vi "Vision1.vi"   [LabVIEW 2016]
uses:
  Campbell!!!4-12/AxonCode/Robot Global Data.vi
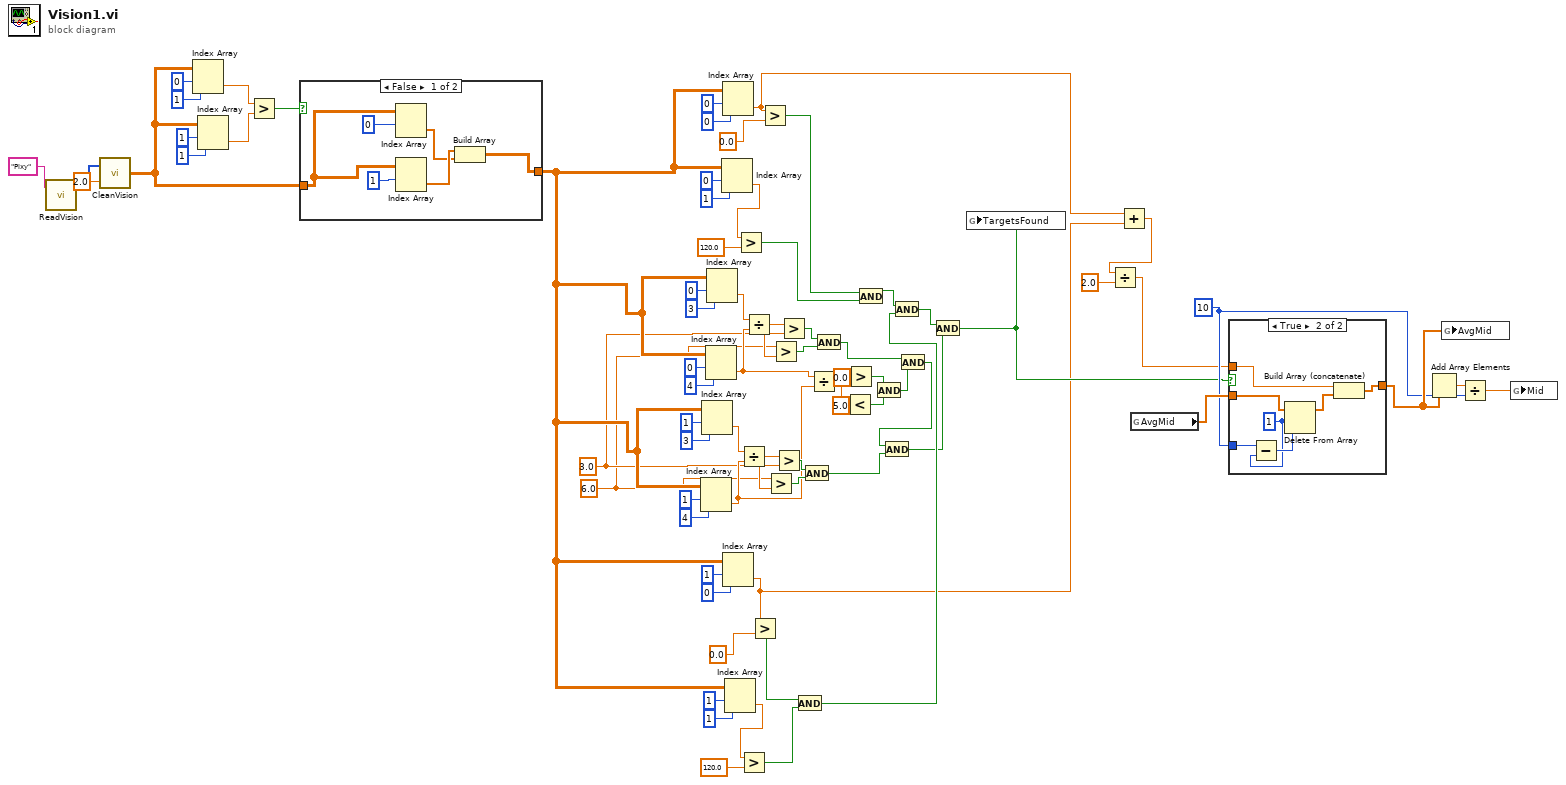
[diagram p0: block diagram]
diagram:
  w1 = 6.0 ("x")
  w2 = 3.0 ("y")
  w58 = 10
  n1 = call "ReadVision.vi"("Name"="Pixy") -> ("Target Data"=w73:u16[])  [unwired: 2 in]
  n2 = call "CleanVision.vi"("Targets"=2.0, "Input"=w73) -> ("Output"=w4:dbl[][])
  n3 = Index Array(array=w4, index (row)=0, index (col)=1 ("disabled index (col)")) -> (element=w6:dbl)
  n4 = Index Array(array=w4, index (row)=1, index (col)=1 ("disabled index (col)")) -> (element=w7:dbl)
  n5 = Greater?(x=w6, y=w7) -> (0:w5:bool)
  n6 = case shown="False" w5 {
    tunnel: w4 -> [w79 w81]
    tunnel: [w75 w81] -> w3
    frame False {
      n7 = Index Array(array=w79, index (row)=0) -> (element=w76:dbl[])  [unwired: 1 in]
      n8 = Index Array(array=w79, index (row)=1) -> (element=w77:dbl[])  [unwired: 1 in]
      n9 = Build Array(w77, w76) -> (w75:dbl[][])
    }
    frame True {
    }
  }
  n10 = Index Array(array=w3, index (row)=1, index (col)=4 ("disabled index (col)")) -> (element=w29:dbl)
  n11 = Index Array(array=w3, index (row)=1, index (col)=3 ("disabled index (col)")) -> (element=w34:dbl)
  n12 = Index Array(array=w3, index (row)=0, index (col)=4 ("disabled index (col)")) -> (element=w30:dbl)
  n13 = Index Array(array=w3, index (row)=0, index (col)=3 ("disabled index (col)")) -> (element=w42:dbl)
  n14 = Index Array(array=w3, index (row)=0, index (col)=1 ("disabled index (col)")) -> (element=w65:dbl)
  n15 = Index Array(array=w3, index (row)=0, index (col)=0 ("disabled index (col)")) -> (element=w13:dbl)
  n16 = Index Array(array=w3, index (row)=1, index (col)=0 ("disabled index (col)")) -> (element=w12:dbl)
  n17 = Index Array(array=w3, index (row)=1, index (col)=1 ("disabled index (col)")) -> (element=w52:dbl)
  n18 = Greater?(x=w65, y=120.0) -> (0:w62:bool)
  n19 = Divide(x=w34, y=w29) -> (x/y=w33:dbl)
  n20 = Greater?(x=w52, y=120.0) -> (0:w49:bool)
  n21 = Divide(x=w42, y=w30) -> (x/y=w41:dbl)
  n22 = Greater?(x=w12, y=0.0) -> (0:w50:bool)
  n23 = Greater?(x=w13, y=0.0) -> (0:w63:bool)
  n24 = Greater?(x=w1, y=w33) -> (0:w31:bool)
  n25 = Greater?(x=w1, y=w41) -> (0:w40:bool)
  n26 = Greater?(x=w33, y=w2) -> (0:w32:bool)
  n27 = Greater?(x=w41, y=w2) -> (0:w39:bool)
  n28 = And(x=w50, y=w49) -> (x .and. y?=w47:bool)
  n29 = And(x=w32, y=w31) -> (x .and. y?=w21:bool)
  n30 = Divide(x=w30, y=w29) -> (x/y=w26:dbl)
  n31 = And(x=w39, y=w40) -> (x .and. y?=w23:bool)
  n32 = Less?(x=w26, y=5.0) -> (x < y?=w24:bool)
  n33 = Greater?(x=w26, y=0.0) -> (0:w25:bool)
  n34 = And(x=w63, y=w62) -> (x .and. y?=w48:bool)
  n35 = And(x=w25, y=w24) -> (x .and. y?=w22:bool)
  n36 = And(x=w48, y=w47) -> (x .and. y?=w18:bool)
  n37 = And(x=w23, y=w22) -> (x .and. y?=w20:bool)
  n38 = And(x=w20, y=w21) -> (x .and. y?=w19:bool)
  n39 = And(x=w18, y=w19) -> (x .and. y?=w17:bool)
  n40 = global write "Robot Global Data.vi" "TargetsFound"(w17) -> ()
  n41 = Add(x=w13, y=w12) -> (x+y=w16:dbl)
  n42 = Divide(x=w16, y=2.0) -> (x/y=w15:dbl)
  n43 = global read "Robot Global Data.vi" "AvgMid"() -> (w60:dbl[])
  n44 = case shown="True" w17 {
    tunnel: w15 -> [_ w89]
    tunnel: [w82 w88] -> w61
    tunnel: w60 -> [w82 w86]
    tunnel: w58 -> [_ w83]
    frame False {
    }
    frame True {
      w84 = 1 ("length")
      n45 = Subtract(x=w83, y=w84) -> (x-y=w85:i32)
      n46 = Delete From Array(array=w86, length=w84, index=w85) -> (array with subset deleted=w87:dbl[])  [unwired: 1 out]
      n47 = Build Array (concatenate)(w89, w87) -> (w88:dbl[])
    }
  }
  n48 = Add Array Elements(numeric array=w61) -> (sum=w69:dbl)
  n49 = global write "Robot Global Data.vi" "AvgMid"(w61) -> ()
  n50 = Divide(x=w69, y=w58) -> (x/y=w59:dbl)
  n51 = global write "Robot Global Data.vi" "Mid"(w59) -> ()
